vi "dfd_Validate Quantization Wls (Easy).vi"(5 "Coef b/v wl":i16=16, 6 "gain setting":cluster{"gain processing":u16, "gain wl":i16}={"gain processing"=0, "gain wl"=16} {"gain processing" items=["On Target", "On Host"]}, 7 "Coef a/k wl":i16=16, 8 "error in (no error)":errorcluster, 11 "filter in":T1={"mSRate_Fs"=1.0, "mSRate_Version"="1.0", "mSRate_Comments"="", "mSRate_OrgCoef"={"type"=enum."Undefined", "gain"=1.0, "coef a (k)"=[], "coef b (v)"=[]}, "mSRate_CurCoef"={"type"=enum."Undefined", "gain"=1.0, "coef a (k)"=[], "coef b (v)"=[]}, "mSRate_Quantized?"=FALSE, "mSRate_QCoef"={"type"=enum."Undefined", "gain"=1.0, "coef a (k)"=[], "coef b (v)"=[]}, "mSRate_QSettings"=[], "mSRate_Order"=0, "mSRate_Scaling"={"mSRate_ScaleByPowerOf2?"=FALSE, "mSRate_ScaleType"=enum."No Norm"}} {"mSRate_QSettings"."source" items=["Coef a/k"=0, "Coef b/v"=7, "Input"=1, "Output"=2, "Multiplicand"=3, "Product"=4, "Sum"=5, "Delay"=6, "Gain"=8]}) -> (0 "error out":errorcluster, 3 "filter out":T1={"mSRate_Fs"=1.0, "mSRate_Version"="1.0", "mSRate_Comments"="", "mSRate_OrgCoef"={"type"=enum."Undefined", "gain"=1.0, "coef a (k)"=[], "coef b (v)"=[]}, "mSRate_CurCoef"={"type"=enum."Undefined", "gain"=1.0, "coef a (k)"=[], "coef b (v)"=[]}, "mSRate_Quantized?"=FALSE, "mSRate_QCoef"={"type"=enum."Undefined", "gain"=1.0, "coef a (k)"=[], "coef b (v)"=[]}, "mSRate_QSettings"=[], "mSRate_Order"=0, "mSRate_Scaling"={"mSRate_ScaleByPowerOf2?"=FALSE, "mSRate_ScaleType"=enum."No Norm"}} {"mSRate_QSettings"."source" items=["Coef a/k"=0, "Coef b/v"=7, "Input"=1, "Output"=2, "Multiplicand"=3, "Product"=4, "Sum"=5, "Delay"=6, "Gain"=8]})   [LabVIEW 2017, in "NI_DigFilter_FXP.lvlib"]
uses:
  <vilib>/addons/Digital Filter Design/NI_DigFilter_FXP.lvlib
  <vilib>/addons/Digital Filter Design/_Objects.llb/DFD Filter Obj.ctl
  <vilib>/addons/Digital Filter Design/_Objects.llb/DFD Filter Coef.ctl
  <vilib>/addons/Digital Filter Design/_Objects.llb/DFD Filter Structure Type Selector.ctl
  <vilib>/addons/Digital Filter Design/_Objects.llb/dfd_Internal Quantization Settings.ctl
  <vilib>/addons/Digital Filter Design/_Objects.llb/dfd_Internal Quantization Srcs.ctl
  <vilib>/addons/Digital Filter Design/_Objects.llb/DFD Coef Norm Type.ctl
  <vilib>/addons/Digital Filter Design/NI_DigFilterLicensed.lvlib
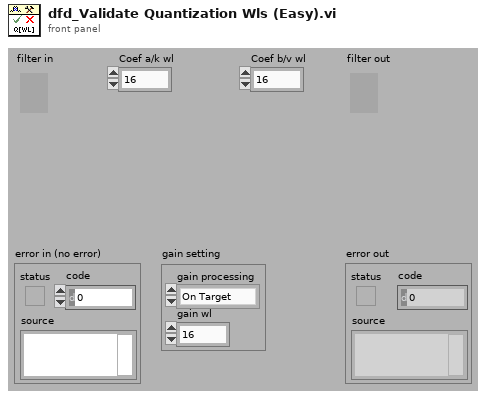
[diagram p1: front panel]
types:
  T1 = typedef "NI_DigFilterLicensed.lvlib/DFD Filter Obj.ctl" = cluster{"mSRate_Fs":dbl, "mSRate_Version":string, "mSRate_Comments":string, "mSRate_OrgCoef":T2, "mSRate_CurCoef":T2, "mSRate_Quantized?":bool, "mSRate_QCoef":T2, "mSRate_QSettings":T4[], "mSRate_Order":i32, "mSRate_Scaling":cluster{"mSRate_ScaleByPowerOf2?":bool, "mSRate_ScaleType":T6}}
  T2 = typedef "NI_DigFilterLicensed.lvlib/DFD Filter Coef.ctl" = cluster{"type":T3, "gain":dbl, "coef a (k)":dbl[], "coef b (v)":dbl[]}
  T3 = typedef "NI_DigFilterLicensed.lvlib/DFD Filter Structure Type Selector.ctl" = enum16{"Undefined", "FIR Direct Form", "FIR Direct Form Transposed", "FIR Symmetric", "FIR Antisymmetric", "IIR Direct Form I", "IIR Direct Form I Transposed", "IIR Direct Form II", "IIR Direct Form II Transposed", "IIR Cascaded Second Order Sections Form I", "IIR Cascaded Second Order Sections Form I Transposed", "IIR Cascaded Second Order Sections Form II", "IIR Cascaded Second Order Sections Form II Transposed", "Lattice Allpass (basic sections)", "Lattice Allpass (one multiplier sections)", "Lattice Allpass (normalized sections)", "Lattice AR (basic sections)", "Lattice AR (one multiplier sections)", "Lattice AR (normalized sections)", "Lattice MA (minimum phase)", "Lattice MA (maximum phase)", "Lattice ARMA (basic sections)", "Lattice ARMA (one multiplier sections)", "Lattice ARMA (normalized sections)"}
  T4 = typedef "NI_DigFilterLicensed.lvlib/dfd_Internal Quantization Settings.ctl" = cluster{"source":T5, "wl":i16, "iwl":i16, "overflow mode":enum16{"Saturation", "Wrap"}, "rounding mode":enum16{"Nearest", "Truncation"}, "signed?":bool}
  T5 = typedef "NI_DigFilterLicensed.lvlib/dfd_Internal Quantization Srcs.ctl" = u16
  T6 = typedef "NI_DigFilterLicensed.lvlib/DFD Coef Norm Type.ctl" = enum16{"No Norm", "Time Domain 1-Norm", "Time Domain 2-Norm", "Time Domain Inf-Norm"}
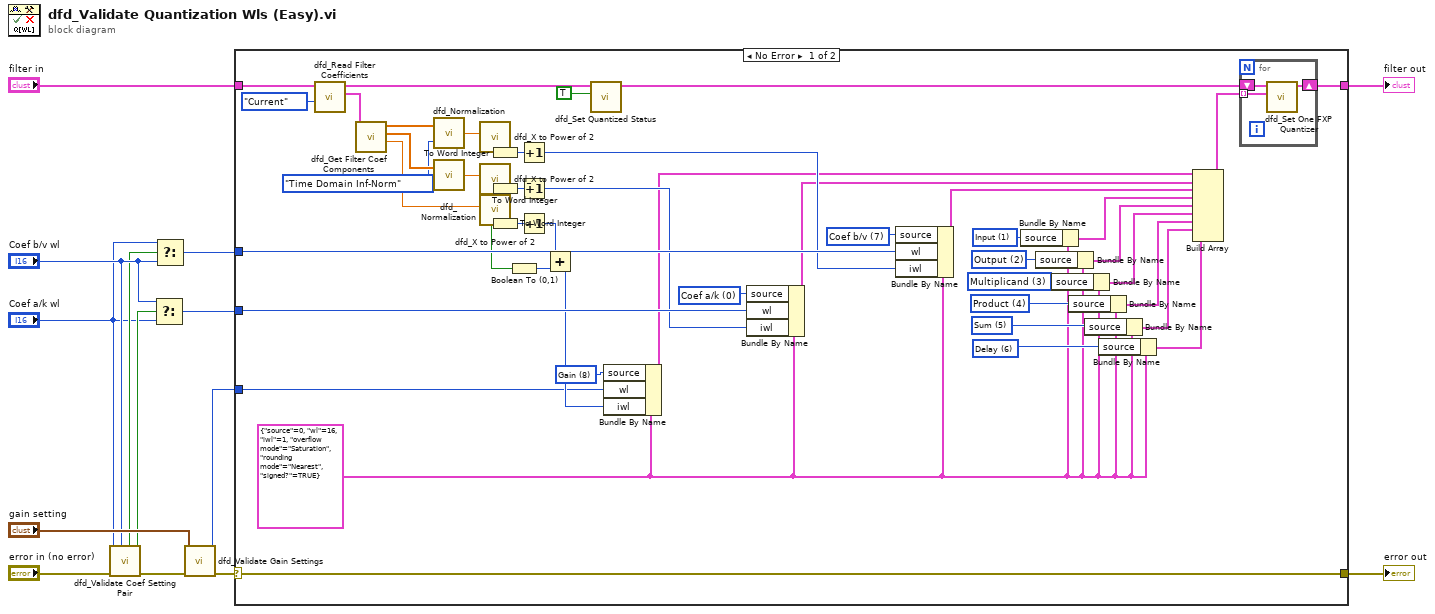
[diagram p0: block diagram]
diagram:
  n1 = call <vilib>:"dfd_Validate Coef Setting Pair.vi"("coef b/v wl"="Coef b/v wl", "error in (no error)"="error in (no error)", "coef a/k wl"="Coef a/k wl") -> ("error out"=w2:errorcluster, "a/k selector"=w4:bool, "b/v selector"=w5:bool)  [unwired: 6 out]
  n2 = Select(t="Coef b/v wl", s=w4, f="Coef a/k wl") -> (s? t:f=w11:i16)
  n3 = Select(t="Coef a/k wl", s=w5, f="Coef b/v wl") -> (s? t:f=w10:i16)
  n4 = call <vilib>:"dfd_Validate Gain Settings.vi"("error in (no error)"=w2, "gain setting"="gain setting") -> ("error out"=w9:errorcluster, "gain wl"=w7:i16)  [unwired: 8 out]
  n5 = case shown="No Error" w9 {
    selector: w9 -> [w38 w68]
    tunnel: [w38 w68] -> w14
    tunnel: "filter in" -> [w63 w67]
    tunnel: [w16 w67] -> w12
    tunnel: w7 -> [w34 _]
    tunnel: w11 -> [w49 _]
    tunnel: w10 -> [w46 _]
    frame No Error {
      w23 = T4 {"source"=0, "wl"=16, "iwl"=1, "overflow mode"=enum."Saturation", "rounding mode"=enum."Nearest", "signed?"=TRUE} ("quantizer")
      w28 = T5 6 items=["Coef a/k"=0, "Coef b/v"=7, "Input"=1, "Output"=2, "Multiplicand"=3, "Product"=4, "Sum"=5, "Delay"=6, "Gain"=8] ("source")
      w29 = T5 5 items=["Coef a/k"=0, "Coef b/v"=7, "Input"=1, "Output"=2, "Multiplicand"=3, "Product"=4, "Sum"=5, "Delay"=6, "Gain"=8] ("source")
      w30 = T5 4 items=["Coef a/k"=0, "Coef b/v"=7, "Input"=1, "Output"=2, "Multiplicand"=3, "Product"=4, "Sum"=5, "Delay"=6, "Gain"=8] ("source")
      w31 = T5 3 items=["Coef a/k"=0, "Coef b/v"=7, "Input"=1, "Output"=2, "Multiplicand"=3, "Product"=4, "Sum"=5, "Delay"=6, "Gain"=8] ("source")
      w32 = T5 2 items=["Coef a/k"=0, "Coef b/v"=7, "Input"=1, "Output"=2, "Multiplicand"=3, "Product"=4, "Sum"=5, "Delay"=6, "Gain"=8] ("source")
      w33 = T5 1 items=["Coef a/k"=0, "Coef b/v"=7, "Input"=1, "Output"=2, "Multiplicand"=3, "Product"=4, "Sum"=5, "Delay"=6, "Gain"=8] ("source")
      w42 = T5 7 items=["Coef a/k"=0, "Coef b/v"=7, "Input"=1, "Output"=2, "Multiplicand"=3, "Product"=4, "Sum"=5, "Delay"=6, "Gain"=8] ("source")
      w47 = T5 0 items=["Coef a/k"=0, "Coef b/v"=7, "Input"=1, "Output"=2, "Multiplicand"=3, "Product"=4, "Sum"=5, "Delay"=6, "Gain"=8] ("source")
      w51 = T5 8 items=["Coef a/k"=0, "Coef b/v"=7, "Input"=1, "Output"=2, "Multiplicand"=3, "Product"=4, "Sum"=5, "Delay"=6, "Gain"=8] ("source")
      w58 = DFD_Coef_Norm_Type."Time Domain Inf-Norm" ("scale type")
      n6 = call <vilib>:"dfd_Read Filter Coefficients.vi"("coef source"=enum16{"Original", "Current", "Quantized"}."Current", "filter in"=w63) -> ("filter coef"=w61:T2, "filter out"=w44:T1)  [unwired: 1 in, 7 out]
      n7 = call <vilib>:"dfd_Get Filter Coef Components.vi"("filter coef"=w61) -> ("gain"=w57:dbl, "coef a (k)"=w59:dbl[], "coef b (v)"=w60:dbl[])  [unwired: 1 in, 7 out]
      n8 = call <vilib>:"dfd_Normalization.vi"("scale type"=w58, "h(n)"=w60) -> ("norm"=w55:dbl)
      n9 = call <vilib>:"dfd_Normalization.vi"("scale type"=w58, "h(n)"=w59) -> ("norm"=w56:dbl)
      n10 = call <vilib>:"dfd_X to Power of 2.vi"("x"=w55) -> ("n"=w54:dbl)  [unwired: 10 out]
      n11 = call <vilib>:"dfd_X to Power of 2.vi"("x"=w56) -> ("n"=w53:dbl)  [unwired: 10 out]
      n12 = call <vilib>:"dfd_X to Power of 2.vi"("x"=w57) -> ("n"=w52:dbl, "is 2^n?"=w35:bool)  [unwired: 9 out]
      n13 = To Word Integer(number=w54) -> (16bit integer=w45:i16)
      n14 = To Word Integer(number=w53) -> (16bit integer=w48:i16)
      n15 = To Word Integer(number=w52) -> (16bit integer=w50:i16)
      n16 = Boolean To (0,1)(Boolean=w35) -> (0, 1=w36:i16)
      n17 = Increment(x=w45) -> (x+1=w41:i16)
      n18 = Increment(x=w48) -> (x+1=w40:i16)
      n19 = Increment(x=w50) -> (x+1=w39:i16)
      n20 = Add(x=w39, y=w36) -> (x+y=w37:i16)
      n21 = call <vilib>:"dfd_Set Quantized Status.vi"("quantized?"=TRUE, "filter in"=w44) -> ("filter out"=w17:T1)  [unwired: 1 in, 8 out]
      n22 = Bundle By Name(cluster=w23, "source"=w51, "wl"=w34, "iwl"=w37) -> (w27:T4)
      n23 = Bundle By Name(cluster=w23, "source"=w47, "wl"=w49, "iwl"=w40) -> (w26:T4)
      n24 = Bundle By Name(cluster=w23, "source"=w42, "wl"=w46, "iwl"=w41) -> (w25:T4)
      n25 = Bundle By Name(cluster=w23, "source"=w33) -> (w24:T4)
      n26 = Bundle By Name(cluster=w23, "source"=w32) -> (w15:T4)
      n27 = Bundle By Name(cluster=w23, "source"=w31) -> (w22:T4)
      n28 = Bundle By Name(cluster=w23, "source"=w30) -> (w21:T4)
      n29 = Bundle By Name(cluster=w23, "source"=w29) -> (w20:T4)
      n30 = Bundle By Name(cluster=w23, "source"=w28) -> (w19:T4)
      n31 = Build Array(w27, w26, w25, w24, w15, w22, w21, w20, w19) -> (w18:T4[])
      n32 = for {
        tunnel: w18 -> [w66] mode=indexing
        shift-right: [w64] -> w16
        shift-left: w17 -> [w65]
        n33 = call <vilib>:"dfd_Set One FXP Quantizer.vi"("quantization settings"=w66, "filter in"=w65) -> ("filter out"=w64:T1)  [unwired: 1 in, 8 out]
      }
    }
    frame Error {
    }
  }
  "filter out" <- w12
  "error out" <- w14
